vi "ROS_MasteR_registerServiceReply.vi"(3 "Service":T1) -> (1 "XML":string)   [LabVIEW 2015]
uses:
  ROS_Service.ctl
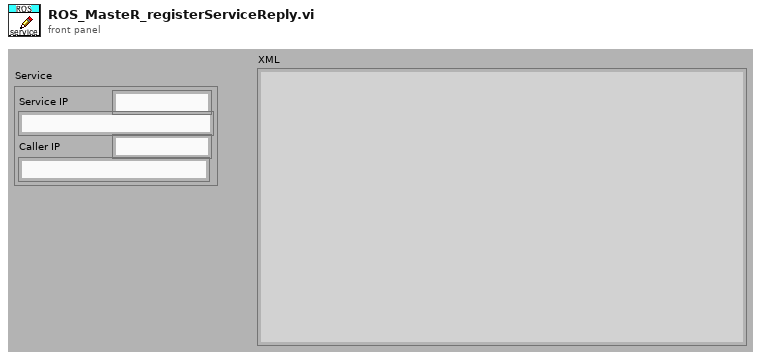
[diagram p1: front panel]
types:
  T1 = typedef "ROS_Service.ctl" = cluster{"Service":string, "Service IP":string, "Caller IP":string, "Caller ID":string}
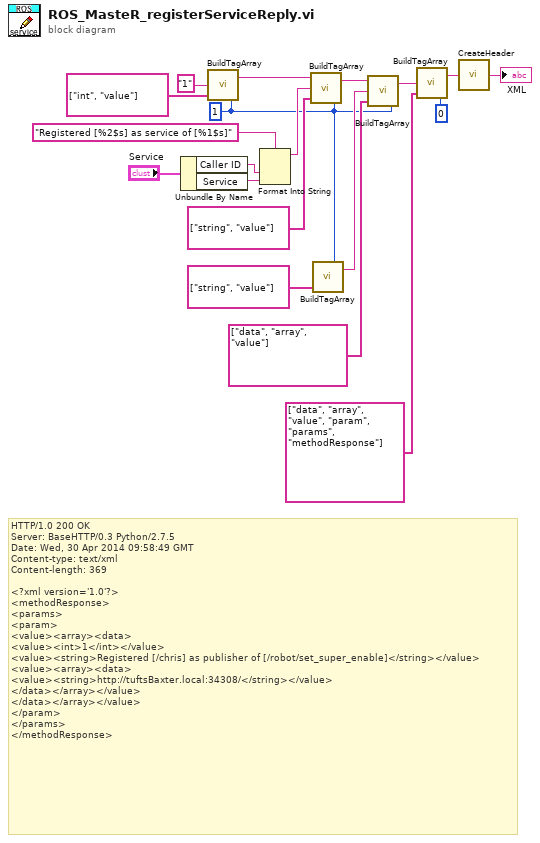
[diagram p0: block diagram]
diagram:
  w1 = i8 1 ("Indent")
  # "HTTP/1.0 200 OK\nServer: BaseHTTP/0.3 Python/2.7.5\nDate: Wed, 30 Apr 2014 09:58:49 GMT\nContent-type: text/xml\nContent-length: 369\n\n<?xml version='1.0'?>\n<methodResponse>\n<params>\n<param>\n<value><array><data>\n<value><int>1</int></value>\n<value><string>Registered [/chris] as publisher of [/robot/set_super_enable]</string></value>\n<value><array><data>\n<value><string>http://tuftsBaxter.local:34308/</string></value>\n</data></array></value>\n</data></array></value>\n</param>\n</params>\n</methodResponse>"
  n1 = Unbundle By Name("Service") -> ("Caller ID"=w16:string, "Service"=w17:string)
  n2 = call "BuildTagArray.vi"("Indent"=w1, "tags"=string[] ["int", "value"], "value"="1") -> ("string out"=w11:string)  [unwired: 1 in]
  n3 = Format Into String(format string="Registered [%2$s] as service of [%1$s]", w16, w17) -> (resulting string=w15:string)  [unwired: 2 in, 1 out]
  n4 = call "BuildTagArray.vi"("Indent"=w1, "tags"=string[] ["string", "value"], "value"=w15, "string in"=w11) -> ("string out"=w10:string)
  n5 = call "BuildTagArray.vi"("Indent"=w1, "tags"=string[] ["string", "value"]) -> ("string out"=w3:string)  [unwired: 2 in]
  n6 = call "BuildTagArray.vi"("Indent"=w1, "tags"=string[] ["data", "array", "value"], "value"=w3, "string in"=w10) -> ("string out"=w9:string)
  n7 = call "BuildTagArray.vi"("Indent"=i8 0, "tags"=string[] ["data", "array", "value", "param", "params", "methodResponse"], "value"=w9) -> ("string out"=w7:string)  [unwired: 1 in]
  n8 = call "CreateHeader.vi"("Content"=w7) -> ("XML"=→"XML":string)
